vi "zad6.vi"(8 "error in (no error)":errorcluster, 11 "N":dbl) -> (0 "Min":dbl, 1 "error out":errorcluster, 2 "Max":dbl, 3 "Œrednia":dbl, 4 "Mediana":dbl, 5 "Odchylenie Stadndardowe":dbl)   [LabVIEW 2017]
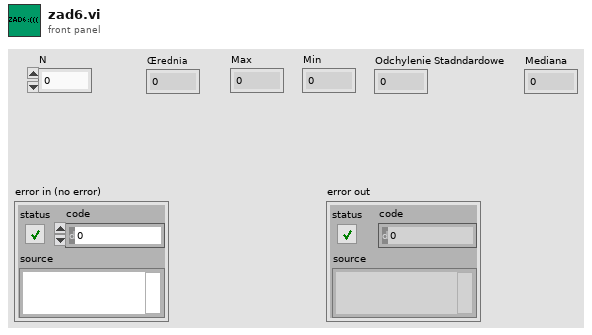
[diagram p1: front panel]
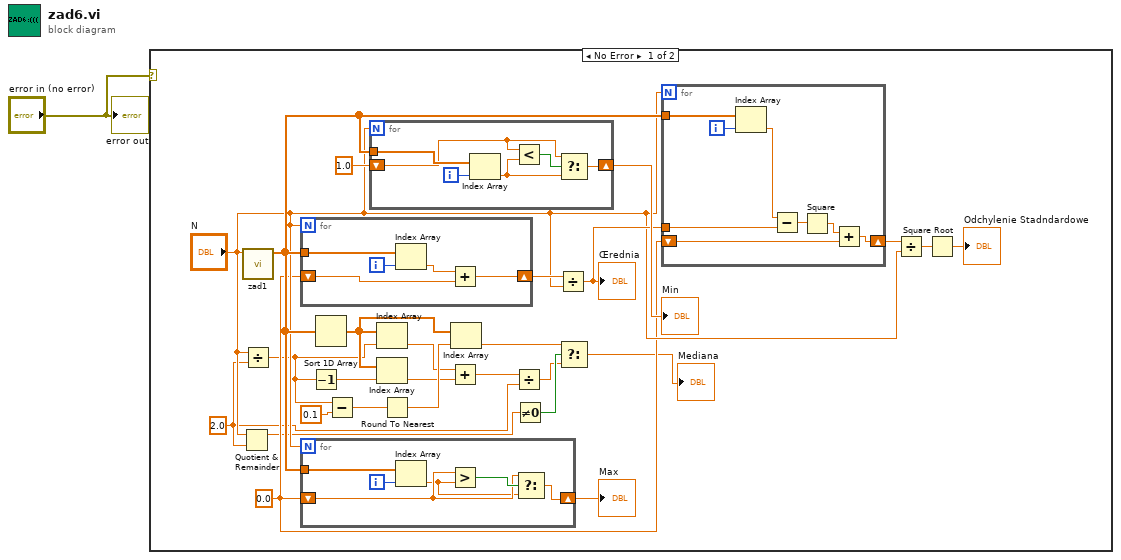
[diagram p0: block diagram]
diagram:
  n1 = case shown="No Error" "error in (no error)" {
    frame No Error {
      w3 = 2.0 ("Numeric")
      w15 = 0.0 ("Numeric")
      n2 = Quotient & Remainder(x="N", y=w3) -> (x-y*floor(x/y)=w14:dbl)  [unwired: 1 out]
      n3 = call "zad1.vi"("Numeric"="N") -> ("Array"=w19:dbl[])  [unwired: 9 in, 1 out]
      n4 = Divide(x="N", y=w3) -> (x/y=w6:dbl)
      n5 = for {
        N: "N" -> [_]
        shift-right: [w51] -> w27
        shift-left: w15 -> [w52]
        tunnel: w19 -> [w49]
        i -> [w50]
        n6 = Index Array(array=w49, index=w50) -> (element=w48:dbl)
        n7 = Add(x=w48, y=w52) -> (x+y=w51:dbl)
      }
      n8 = for {
        N: "N" -> [_]
        tunnel: w19 -> [w47]
        shift-right: [w45] -> w26
        shift-left: w15 -> [w43]
        i -> [w46]
        n9 = Index Array(array=w47, index=w46) -> (element=w42:dbl)
        n10 = Greater?(x=w43, y=w42) -> (0:w44:bool)
        n11 = Select(t=w43, s=w44, f=w42) -> (s? t:f=w45:dbl)
      }
      "Max" <- w26
      n12 = Decrement(x=w6) -> (x-1=w7:dbl)
      n13 = Sort 1D Array(array=w19) -> (sorted array=w8:dbl[])
      n14 = Subtract(x=w6, y=0.1 ("Numeric")) -> (x-y=w13:dbl)
      n15 = for {
        N: "N" -> [_]
        tunnel: w19 -> [w41]
        shift-right: [w39] -> w25
        shift-left: 1.0 ("Numeric") -> [w37]
        i -> [w40]
        n16 = Index Array(array=w41, index=w40) -> (element=w36:dbl)
        n17 = Less?(x=w37, y=w36) -> (x < y?=w38:bool)
        n18 = Select(t=w37, s=w38, f=w36) -> (s? t:f=w39:dbl)
      }
      "Min" <- w25
      n19 = Index Array(array=w8, index=w6) -> (element=w10:dbl)
      n20 = Index Array(array=w8, index=w7) -> (element=w9:dbl)
      n21 = Round To Nearest(number=w13) -> (nearest integer value=w11:dbl)
      n22 = Add(x=w10, y=w9) -> (x+y=w4:dbl)
      n23 = Index Array(array=w8, index=w11) -> (element=w16:dbl)
      n24 = Divide(x=w4, y=w3) -> (x/y=w5:dbl)
      n25 = Not Equal To 0?(x=w14) -> (x != 0?=w17:bool)
      n26 = Divide(x=w27, y="N") -> (x/y=w23:dbl)
      "Œrednia" <- w23
      n27 = Select(t=w16, s=w17, f=w5) -> (s? t:f=→"Mediana":dbl)
      n28 = for {
        N: "N" -> [_]
        shift-right: [w30] -> w22
        shift-left: w15 -> [w31]
        tunnel: w19 -> [w35]
        tunnel: w23 -> [w32]
        i -> [w34]
        n29 = Index Array(array=w35, index=w34) -> (element=w33:dbl)
        n30 = Subtract(x=w33, y=w32) -> (x-y=w29:dbl)
        n31 = Square(x=w29) -> (x^2=w28:dbl)
        n32 = Add(x=w28, y=w31) -> (x+y=w30:dbl)
      }
      n33 = Divide(x=w22, y="N") -> (x/y=w21:dbl)
      n34 = Square Root(x=w21) -> (sqrt(x)=→"Odchylenie Stadndardowe":dbl)
    }
    frame Error {
    }
  }
  "error out" <- "error in (no error)"
